vi "ELOG_AggregationPeriod_Get.vi"(8 "error in (no error)":errorcluster, 11 "OXY_SCPI Reseource In":refnum<visa-resource-name>) -> (0 "error out":errorcluster, 1 "communication_data":T1, 2 "Period duration":dbl, 3 "OXY_SCPI Reseource Out":refnum<visa-resource-name>)   [LabVIEW 2018, in "OXYGEN.lvlib"]
doc: "Queries the numeric data aggregation time for output (in seconds)"
uses:
  OXYGEN.lvlib
  TypeDefs/Cluster_RawCommData.ctl
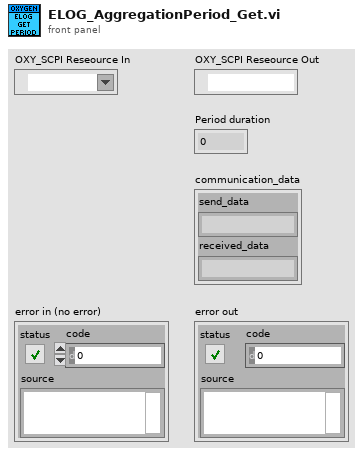
[diagram p1: front panel]
types:
  T1 = typedef "OXYGEN.lvlib/Cluster_RawCommData.ctl" = cluster{"send_data":string, "received_data":string}
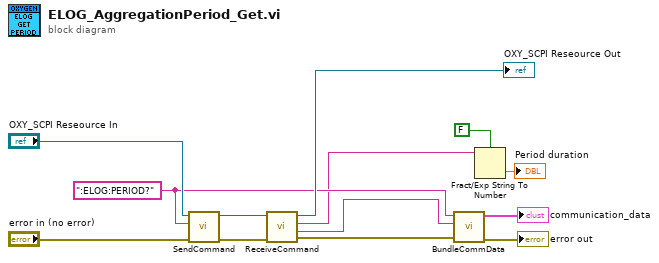
[diagram p0: block diagram]
diagram:
  w5 = ":ELOG:PERIOD?" ("String to Send")
  n1 = call "SendCommand.vi"("error in (no error)"="error in (no error)", "String to Send"=w5, "OXY_SCPI Reseource In"="OXY_SCPI Reseource In") -> ("error out"=w13:errorcluster, "OXY_SCPI Reseource Out"=w12:refnum<visa-resource-name>)  [unwired: 7 in]
  n2 = call "ReceiveCommand.vi"("error in (no error)"=w13, "OXY_SCPI Reseource In"=w12) -> ("error out"=w4:errorcluster, "received Data with Header"=w6:string, "received Data"=w3:string, "OXY_SCPI Reseource Out"=→"OXY_SCPI Reseource Out":refnum<visa-resource-name>)  [unwired: 6 in]
  n3 = call "BundleCommData.vi"("error in (no error)"=w4, "received_data"=w6, "send_data"=w5) -> ("error out"=→"error out":errorcluster, "communication_data"=→"communication_data":T1)  [unwired: 7 in]
  n4 = Fract/Exp String To Number(use system decimal point (T)=FALSE, string=w3) -> (number=→"Period duration":dbl)  [unwired: 2 in, 1 out]
